vi "Read Bus Monitor Log.vi"(8 "error in (no error)":errorcluster, 11 "1553 Component in":refnum<class "1553 Component.lvclass">) -> (0 "error out":errorcluster, 1 "Bus B Monitor Log":string[][](array[string]), 2 "Bus A Monitor Log":string[][](array[string]), 3 "1553 Component out":refnum<class "1553 Component.lvclass">)   [LabVIEW 2016, in "BCI-1553 API.lvlib" / "1553 Component.lvclass"]
doc: "Read the current log stored by the bus monitor for both Bus A and Bus B. Depending on the data rates in the system, these logs may roll-over at various times in the application execution."
uses:
  1553 Component.lvclass
  Bus Monitor/Bus Monitor.lvclass
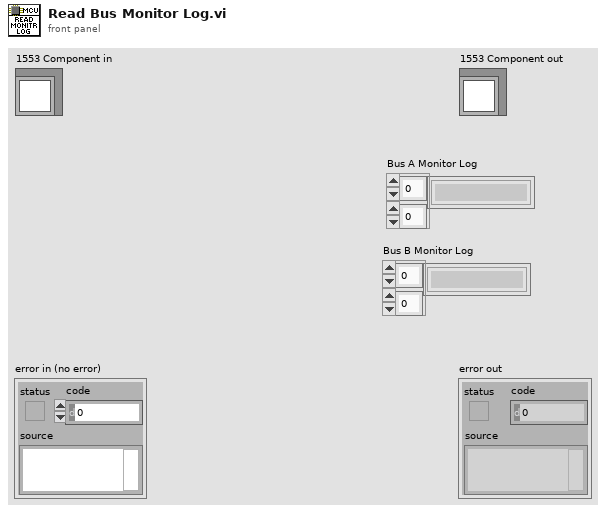
[diagram p1: front panel]
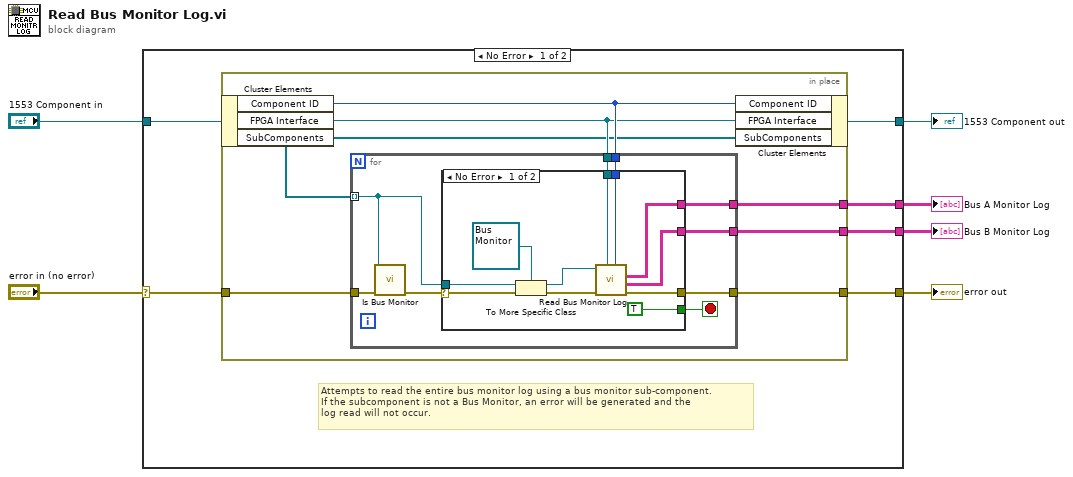
[diagram p0: block diagram]
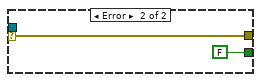
[diagram p2: hidden frame]
diagram:
  n1 = case shown="No Error" "error in (no error)" {
    selector: "error in (no error)" -> [w10 w43]
    tunnel: [w9 w43] -> w4
    tunnel: [w11 w42] -> w3
    tunnel: "1553 Component in" -> [w12 w42]
    tunnel: [w8 _] -> w2
    tunnel: [w7 _] -> w1
    frame No Error {
      # "Attempts to read the entire bus monitor log using a bus monitor sub-component.\nIf the subcomponent is not a Bus Monitor, an error will be generated and the\nlog read will not occur."
      n2 = in-place {
        in-place-border: w10 -> [w17]
        in-place-border: [w16] -> w9
        in-place-border: [w15] -> w8
        in-place-border: [w14] -> w7
        n3 = in-place-cluster #1(w12) -> ("Component ID"=w19:u8, "FPGA Interface"=w18:refnum<class "FPGA Interface.lvclass">, "SubComponents"=w13:refnum<class "1553 SubComponent.lvclass">[])
        n4 = for {
          tunnel: w13 -> [w24] mode=indexing
          tunnel: w19 -> [w28]
          tunnel: w18 -> [w27]
          tunnel: w17 -> [w23]
          tunnel: [w26] -> w16
          tunnel: [w21] -> w15
          tunnel: [w20] -> w14
          stop <- w25 stop-if-true
          n5 = call "Is Bus Monitor.vi"("error in (no error)"=w23, "1553 SubComponent"=w24) -> ("error out"=w22:errorcluster)  [unwired: 9 in]
          n6 = case shown="No Error" w22 {
            selector: w22 -> [w37 w41]
            tunnel: w28 -> [w32 _]
            tunnel: w27 -> [w33 _]
            tunnel: [w31 w41] -> w26
            tunnel: w24 -> [w38 _]
            tunnel: [TRUE FALSE] -> w25
            tunnel: [w30 _] -> w21
            tunnel: [w29 _] -> w20
            frame No Error {
              n7 = To More Specific Class(target class=refnum<class "Bus Monitor.lvclass"> refnum ("BCI-1553 API.lvlib:Bus Monitor.lvclass"), reference=w38, error in=w37) -> (specific class reference=w35:refnum<class "Bus Monitor.lvclass">, error out=w34:errorcluster)
              n8 = call-dynamic "Read Bus Monitor Log.vi"("Component ID"=w32, "FPGA Interface"=w33, "error in (no error)"=w34, "Bus Monitor in"=w35) -> ("error out"=w31:errorcluster, "Bus B Monitor Log"=w29:string[][], "Bus A Monitor Log"=w30:string[][])  [unwired: 4 in, 1 out]
            }
            frame Error {
            }
          }
        }
        n9 = in-place-cluster #1("Component ID"=w19, "FPGA Interface"=w18, "SubComponents"=w13) -> (w11:refnum<class "1553 Component.lvclass">)
      }
    }
    frame Error {
    }
  }
  "error out" <- w4
  "1553 Component out" <- w3
  "Bus A Monitor Log" <- w2
  "Bus B Monitor Log" <- w1
